vi "SetHSL.vi"(0 "ColorHLS in":refnum<class "ColorHSL.lvclass">, 5 "H":u8, 7 "L":u8, 9 "S":u8, 11 "error in (no error)":errorcluster) -> (4 "ColorHLS out":refnum<class "ColorHSL.lvclass">, 15 "error out":errorcluster)   [LabVIEW 2021, in "Picture2D.lvlib" / "ColorHSL.lvclass"]
uses:
  ColorHSL.lvclass
  ColorHSL.lvclass/ColorHSL.ctl
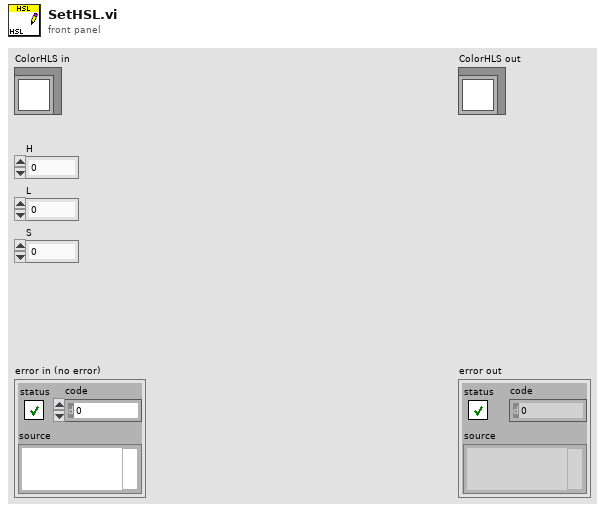
[diagram p1: front panel]
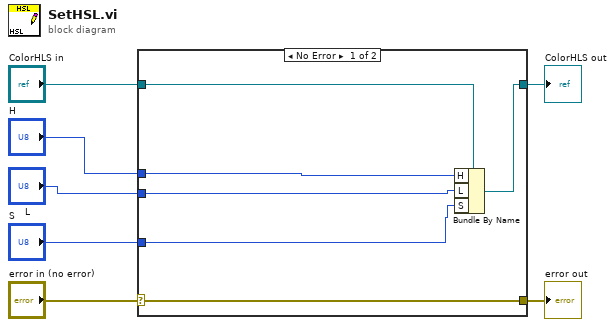
[diagram p0: block diagram]
diagram:
  n1 = case shown="No Error" "error in (no error)" {
    selector: "error in (no error)" -> [w13 w14]
    tunnel: [w13 w14] -> w6
    tunnel: [w11 w15] -> w4
    tunnel: "ColorHLS in" -> [w12 w15]
    tunnel: "H" -> [w10 _]
    tunnel: "L" -> [w9 _]
    tunnel: "S" -> [w8 _]
    frame No Error {
      n2 = Bundle By Name(cluster=w12, "H"=w10, "L"=w9, "S"=w8) -> (w11:refnum<class "ColorHSL.lvclass">)
    }
    frame Error {
    }
  }
  "error out" <- w6
  "ColorHLS out" <- w4
